vi "Format Client MQTT Topics.vi"(10 "Topics Strings":string[](array[string]), 11 "Module ID":i32) -> (3 "Topics":string[](array[string]))   [LabVIEW 2020, in "MQTT_Client.lvlib"]
uses:
  MQTT_Client.lvlib
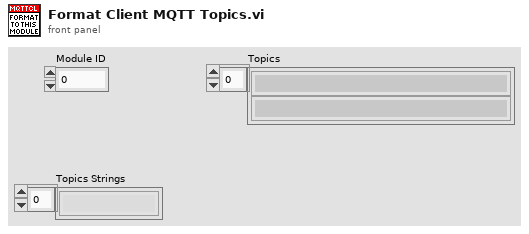
[diagram p1: front panel]
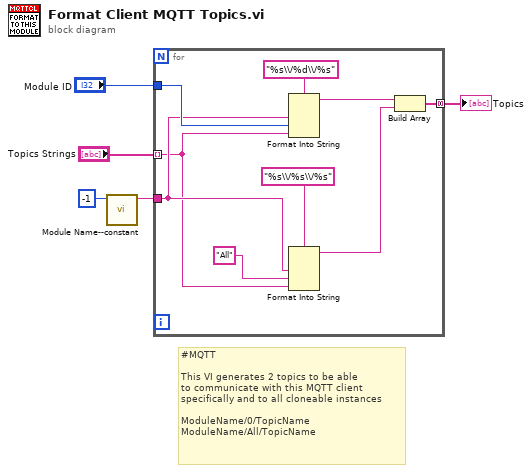
[diagram p0: block diagram]
diagram:
  # "#MQTT  \n\nThis VI generates 2 topics to be able\nto communicate with this MQTT client\nspecifically and to all cloneable instances\n\nModuleName/0/TopicName\nModuleName/All/TopicName"
  n1 = call "Module Name--constant.vi"("Module ID"=-1) -> ("Module Name"=w2:string)  [unwired: 10 in]
  n2 = for {
    tunnel: "Module ID" -> [w14]
    tunnel: [w8] -> w3 mode=concatenating
    tunnel: w2 -> [w7]
    tunnel: "Topics Strings" -> [w6] mode=indexing
    n3 = Format Into String(format string="%s\\/%d\\/%s", w7, w14, w6) -> (resulting string=w10:string)  [unwired: 2 in, 1 out]
    n4 = Format Into String(format string="%s\\/%s\\/%s", w7, "All" ("input 2"), w6) -> (resulting string=w9:string)  [unwired: 2 in, 1 out]
    n5 = Build Array(w10, w9) -> (w8:string[])
  }
  "Topics" <- w3
